vi "运维调试_古田污水厂.vi"() -> ()   [LabVIEW 2016]
uses:
  <vilib>/Utility/miscctls.llb/LVPointTypeDef.ctl
  API/CodCr/CodCr.lvlib
  PLC/PLC.lvlib
panel:
  in  "运维调试单选按钮":enum32{"采配水", "CodCr", "总磷氨氮", "pH", "其他"}(xcontrol)
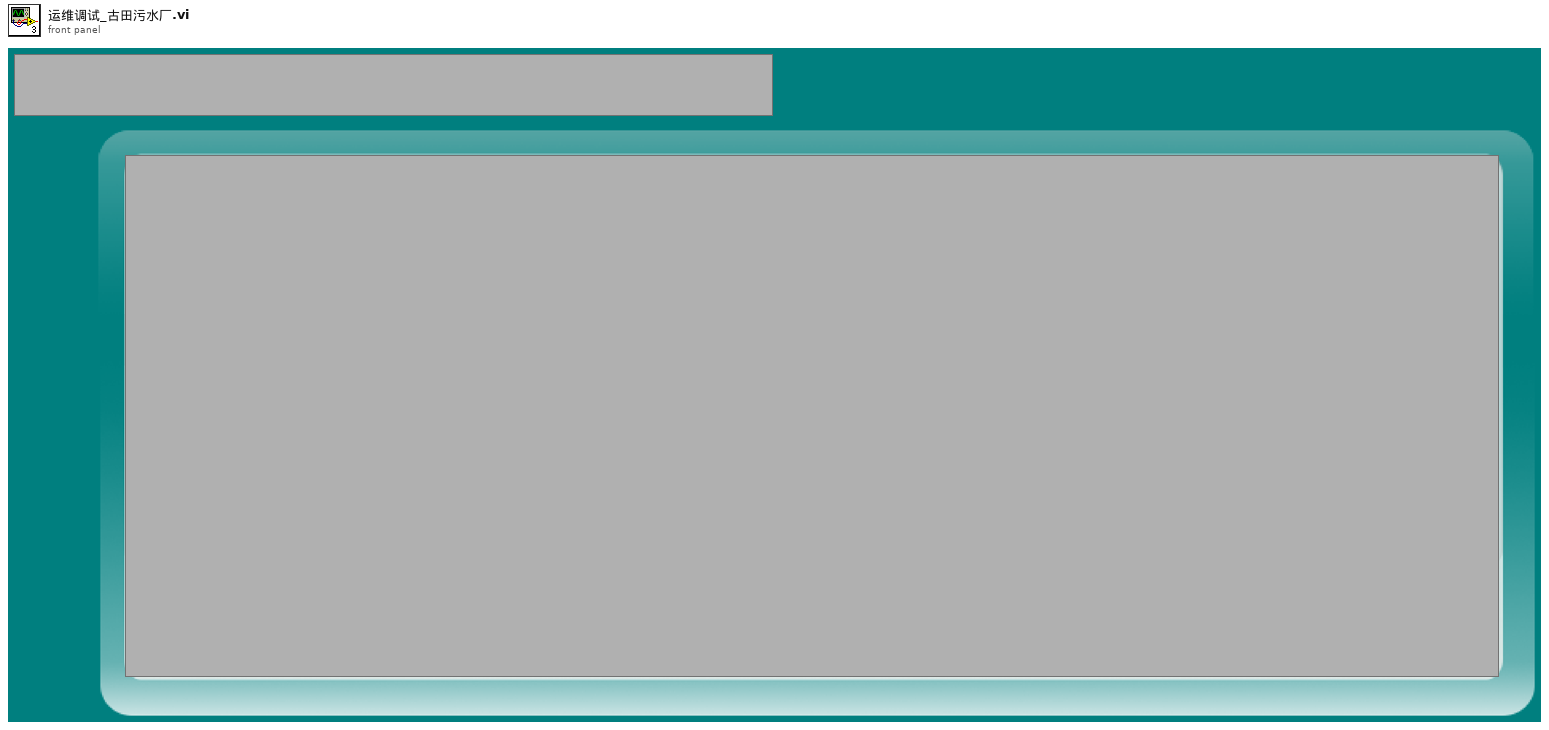
[diagram p1: front panel]
types:
  T1 = typedef "LVPointTypeDef.ctl" = cluster{"Horizontal":i16, "Vertical":i16}
  T2 = enum32{"Bad", "Idle", "Run top level", "Running"}
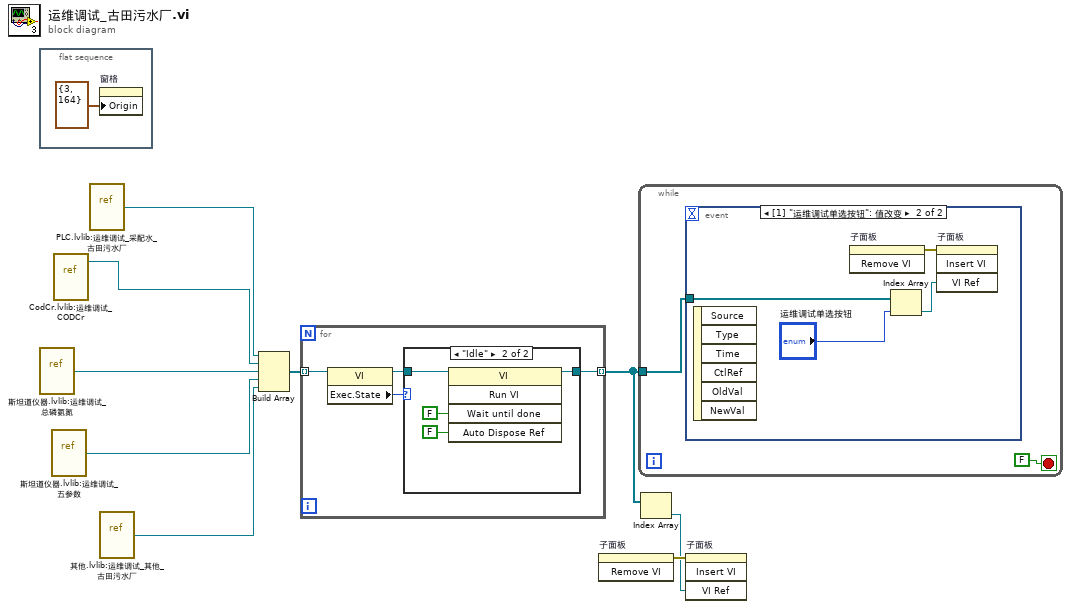
[diagram p0: block diagram]
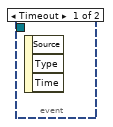
[diagram p3: hidden frame]
diagram:
  n1 = flat-sequence {
    frame #0 {
      n2 = property on="窗格" class="Pane"("Origin"=T1 {"Horizontal"=3, "Vertical"=164} ("原点")) -> ()  [unwired: 2 in, 2 out]
    }
  }
  n3 = vi-ref "斯坦道仪器.lvlib:运维调试_总磷氨氮.vi"() -> (w3:refnum<vi>)
  n4 = vi-ref "斯坦道仪器.lvlib:运维调试_五参数.vi"() -> (w5:refnum<vi>)
  n5 = vi-ref "CodCr.lvlib:运维调试_CODCr.vi"() -> (w1:refnum<vi>)
  n6 = vi-ref "PLC.lvlib:运维调试_采配水_古田污水厂.vi"() -> (w6:refnum<vi>)
  n7 = vi-ref "其他.lvlib:运维调试_其他_古田污水厂.vi"() -> (w2:refnum<vi>)
  n8 = Build Array(w6, w1, w3, w5, w2) -> (w4:refnum<vi>[])
  n9 = for {
    tunnel: w4 -> [w14] mode=indexing
    tunnel: [w11] -> w8 mode=indexing
    n10 = property class="VI"(reference=w14) -> (reference out=w12:refnum<vi>, "Exec.State"=w13:T2)  [unwired: 1 in, 1 out]
    n11 = case shown="\"Idle\"" w13 {
      tunnel: w12 -> [w15 w17]
      tunnel: [w15 w16] -> w11
      frame "Bad", Default {
      }
      frame "Idle" {
        n12 = invoke class="VI" method="Run VI"(reference=w17, "Wait until done"=FALSE ("结束前等待"), "Auto Dispose Ref"=FALSE ("自动销毁引用")) -> (reference out=w16:refnum<vi>)  [unwired: 2 in, 4 out]
      }
    }
  }
  n13 = invoke on="子面板" class="SubPnl" method="Remove VI"() -> (error out=w9:errorcluster)  [unwired: 3 in, 2 out]
  n14 = while {
    tunnel: w8 -> [w20]
    stop <- FALSE stop-if-true
    n15 = event shown="[1] \"运维调试单选按钮\": 值改变" {
      selector: _ -> [_ _]
      dyn-events: _ -> [_ _]
      timeout: _ -> [_ _]
      tunnel: w20 -> [_ w23]
      event Timeout {
        n16 = event-data() -> ()  [unwired: 1 in, 3 out]
      }
      event "运维调试单选按钮": Value Change {
        n17 = event-data() -> ()  [unwired: 1 in, 6 out]
        n18 = invoke on="子面板" class="SubPnl" method="Remove VI"() -> (error out=w25:errorcluster)  [unwired: 3 in, 2 out]
        n19 = Index Array(array=w23, index="运维调试单选按钮") -> (element=w22:refnum<vi>)
        n20 = invoke on="子面板" class="SubPnl" method="Insert VI"(error in=w25, "VI Ref"=w22) -> ()  [unwired: 2 in, 4 out]
      }
    }
  }
  n21 = Index Array(array=w8) -> (element=w7:refnum<vi>)  [unwired: 1 in]
  n22 = invoke on="子面板" class="SubPnl" method="Insert VI"(error in=w9, "VI Ref"=w7) -> ()  [unwired: 2 in, 4 out]
